vi "User_Regist.vi"() -> ()   [LabVIEW 2020]
panel:
  in  "User_Right":u16(ring) caption="权        限" items=["管理员", "操作员"]
  in  "Confirm Password":string caption="确认密码"
  in  "New Password":string caption="密        码"
  in  "Ok":bool
  in  "User_Name":string caption="用  户  名"
  # "用户注册"
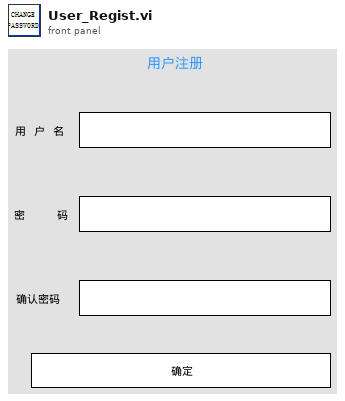
[diagram p1: front panel]
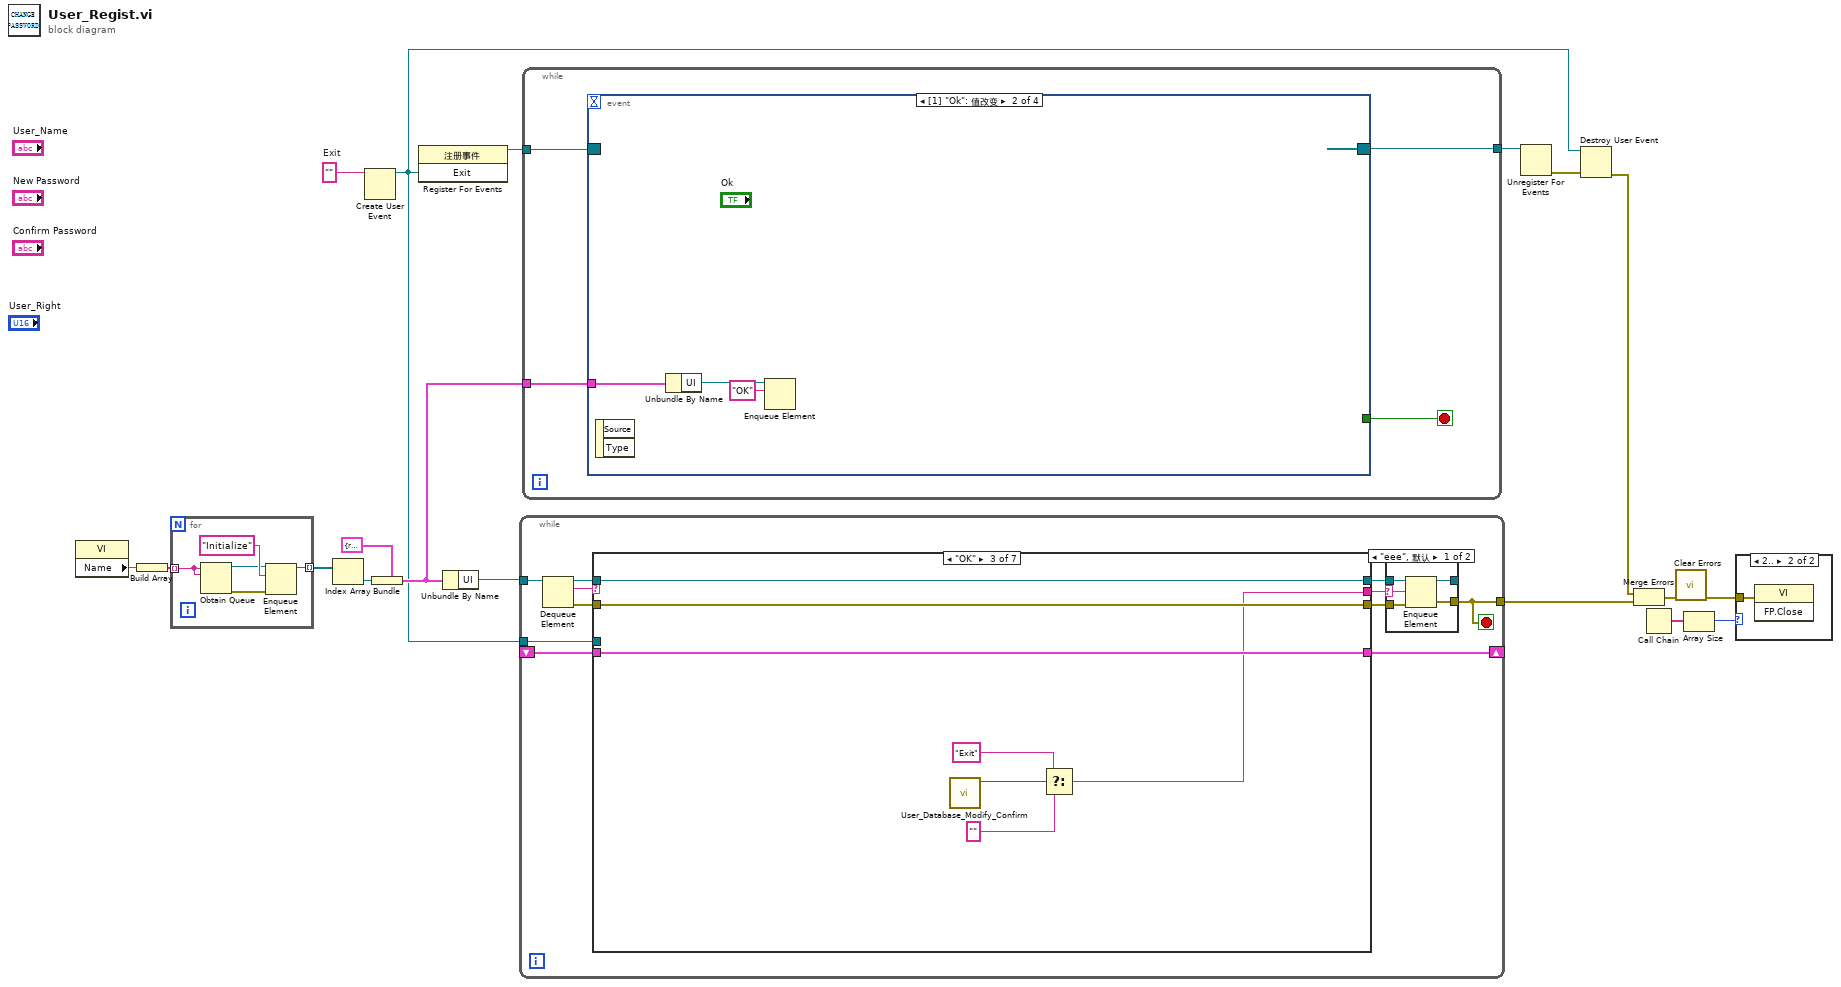
[diagram p0: block diagram]
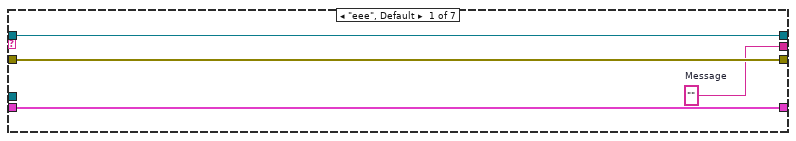
[diagram p4: hidden frame]
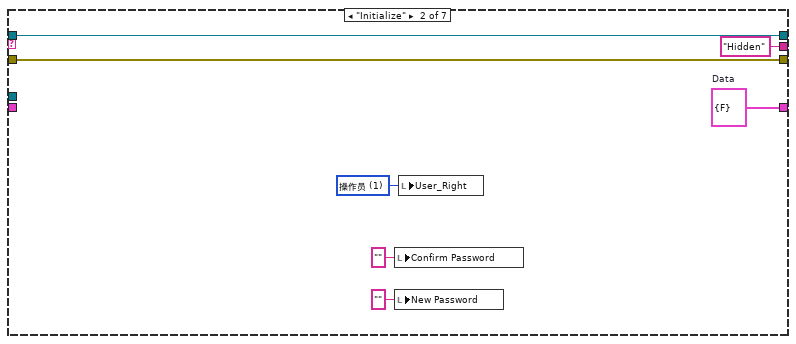
[diagram p5: hidden frame]
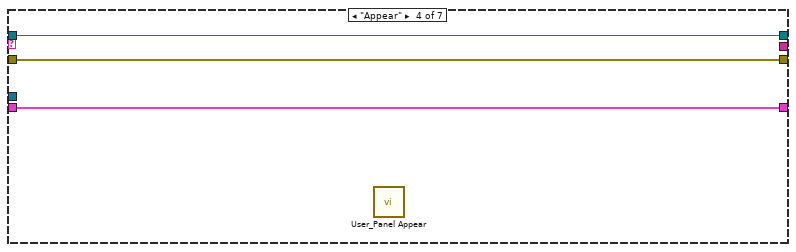
[diagram p6: hidden frame]
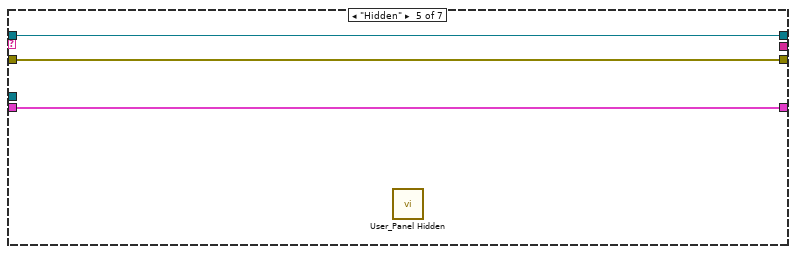
[diagram p7: hidden frame]
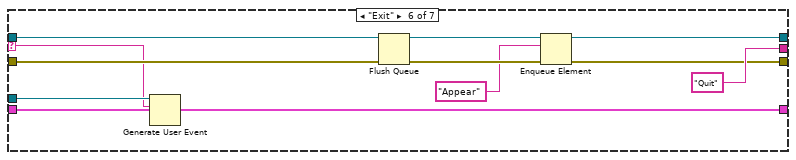
[diagram p8: hidden frame]
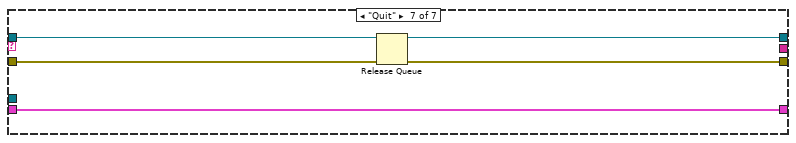
[diagram p9: hidden frame]
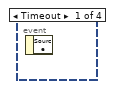
[diagram p10: hidden frame]
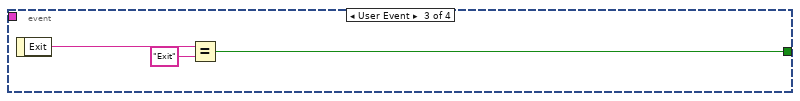
[diagram p11: hidden frame]
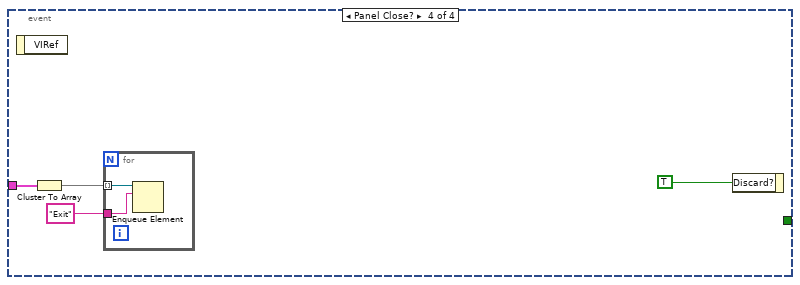
[diagram p12: hidden frame]
diagram:
  w4 = ""  # Exit
  n1 = property class="VI"() -> ("Name"=w14:string)  [unwired: 2 in, 2 out]
  n2 = Build Array(w14) -> (w15:string[])
  n3 = for {
    tunnel: w15 -> [w19] mode=indexing
    tunnel: [w20] -> w9 mode=indexing
    n4 = Obtain Queue(name (unnamed)=w19, element data type=w19) -> (queue out=w22:refnum<queue>, error out=w21:errorcluster)  [unwired: 3 in, 1 out]
    n5 = Enqueue Element(queue=w22, element="Initialize" ("元素"), error in (no error)=w21) -> (queue out=w20:refnum<queue>)  [unwired: 1 in, 2 out]
  }
  n6 = Index Array(array=w9) -> (element=w12:refnum<queue>)  [unwired: 1 in]
  n7 = Create User Event(user event datatype=w4) -> (user event=w8:refnum<user-event>)  [unwired: 1 in, 1 out]
  n8 = Bundle(cluster=cluster{"UI":refnum<queue>} {"UI"=refnum}, "UI"=w12) -> (w13:cluster{"UI":refnum<queue>})
  n9 = register-events(w8) -> (reference out=w5:refnum<event-registration>)  [unwired: 2 in, 1 out]
  n10 = Unbundle By Name(w13) -> ("UI"=w10:refnum<queue>)
  n11 = while {
    tunnel: w10 -> [w34]
    tunnel: [w24] -> w17
    shift-right: [w28] -> _
    shift-left: _ -> [w27]
    tunnel: w8 -> [w26]
    stop <- w24 stop-if-true
    n12 = Dequeue Element(queue=w34) -> (queue out=w33:refnum<queue>, element=w25:string, error out=w30:errorcluster)  [unwired: 2 in, 1 out]
    n13 = case shown="\"OK\"" w25 {
      selector: w25 -> [_ _ _ _ _ w71 _]
      tunnel: w33 -> [w45 w52 w59 w62 w65 w74 w80]
      tunnel: [w45 w52 w59 w62 w65 w66 w80] -> w32
      tunnel: [w44 w51 w58 w61 w64 w67 w77] -> w31
      tunnel: w30 -> [w44 w51 w58 w61 w64 w73 w79]
      tunnel: [w43 "Hidden" ("Message") w53 _ _ "Quit" ("Message") _] -> w29
      tunnel: [w42 w50 w57 w60 w63 w76 w78] -> w28
      tunnel: w27 -> [w42 _ w57 w60 w63 w76 w78]
      tunnel: w26 -> [_ _ _ _ _ w72 _]
      frame "eee", Default {
        w43 = ""  # Message
      }
      frame "Initialize" {
        w48 = u16 1 items=["管理员", "操作员"] ("User_Right")
        w50 = cluster{"Data":bool} {"Data"=FALSE}  # Data
        n14 = local write "Confirm Password"("" ("Confirm Password")) -> ()
        n15 = local write "New Password"("" ("New Password")) -> ()
        n16 = local write "User_Right"(w48) -> ()
      }
      frame "OK" {
        n17 = call "User_Database_Modify_Confirm.vi"() -> ("OK"=w56:bool)  [unwired: 10 in, 1 out]
        n18 = Select(t="Exit", s=w56, f="") -> (s? t:f=w53:string)
      }
      frame "Appear" {
        n19 = call "User_Panel Appear.vi"() -> ()  [unwired: 11 in, 1 out]
      }
      frame "Hidden" {
        n20 = call "User_Panel Hidden.vi"() -> ()  [unwired: 11 in, 1 out]
      }
      frame "Exit" {
        n21 = Generate User Event(user event=w72, event data cluster=w71) -> ()  [unwired: 2 in, 2 out]
        n22 = Flush Queue(queue=w74, error in (no error)=w73) -> (queue out=w70:refnum<queue>, error out=w69:errorcluster)  [unwired: 1 out]
        n23 = Enqueue Element(queue=w70, element="Appear" ("元素"), error in (no error)=w69) -> (queue out=w66:refnum<queue>, error out=w67:errorcluster)  [unwired: 1 in, 1 out]
      }
      frame "Quit" {
        n24 = Release Queue(queue=w80, error in (no error)=w79) -> (error out=w77:errorcluster)  [unwired: 1 in, 2 out]
      }
    }
    n25 = case shown="\"eee\", 默认" w29 {
      selector: w29 -> [w35 _]
      tunnel: w32 -> [w39 w41]
      tunnel: w31 -> [w38 w40]
      tunnel: [w37 w40] -> w24
      tunnel: [w36 w41] -> _
      frame "eee", Default {
        n26 = Enqueue Element(queue=w39, element=w35, error in (no error)=w38) -> (queue out=w36:refnum<queue>, error out=w37:errorcluster)  [unwired: 1 in, 1 out]
      }
      frame "" {
      }
    }
  }
  n27 = while {
    tunnel: w5 -> [w83]
    tunnel: [w82] -> w7
    tunnel: w13 -> [w81]
    stop <- w84 stop-if-true
    n28 = event shown="[1] \"Ok\": 值改变" {
      selector: w83 -> [_ _ _ _]
      dyn-events: [_ _ _ _] -> w82
      timeout: _ -> [_ _ _ _]
      tunnel: [_ _ w89 _] -> w84
      tunnel: w81 -> [_ w87 _ w93]
      event Timeout {
        n29 = event-data() -> ()  [unwired: 1 in, 1 out]
      }
      event "Ok": Value Change {
        n30 = event-data() -> ()  [unwired: 1 in, 2 out]
        n31 = Unbundle By Name(w87) -> ("UI"=w86:refnum<queue>)
        n32 = Enqueue Element(queue=w86, element="OK" ("元素")) -> ()  [unwired: 2 in, 3 out]
      }
      event User Event {
        n33 = event-data() -> ("Exit"=w90:string)  [unwired: 1 in]
        n34 = Equal?(x=w90, y="Exit") -> (x = y?=w89:bool)
      }
      event Panel Close? {
        n35 = event-data() -> ()  [unwired: 1 in, 1 out]
        n36 = Cluster To Array(cluster=w93) -> (array=w92:refnum<queue>[])
        n37 = for {
          tunnel: w92 -> [w96] mode=indexing
          tunnel: "Exit" ("元素") -> [w95]
          n38 = Enqueue Element(queue=w96, element=w95) -> ()  [unwired: 2 in, 3 out]
        }
        n39 = event-data("Discard?"=TRUE ("放弃？")) -> ()  [unwired: 1 in, 1 out]
      }
    }
  }
  n40 = Unregister For Events(event registration refnum=w7) -> (error out=w6:errorcluster)  [unwired: 1 in]
  n41 = Destroy User Event(user event=w8, error in=w6) -> (error out=w16:errorcluster)
  n42 = Merge Errors(w16, w17) -> (w18:errorcluster)
  n43 = Call Chain() -> (call chain=w2:string[])
  n44 = call <vilib>:"Clear Errors.vi"("error in (no error)"=w18) -> ("error out"=w3:errorcluster)  [unwired: 5 in, 1 out]
  n45 = Array Size(array=w2) -> (size(s)=w1:i32)
  n46 = case shown="2.." w1 {
    tunnel: w3 -> [_ w97]
    frame 0, Default {
    }
    frame 2.. {
      n47 = invoke class="VI" method="FP.Close"(error in=w97) -> ()  [unwired: 2 in, 3 out]
    }
  }
